vi "3_Axis_magmeter_MAIN.vi"() -> ()   [LabVIEW 2013]
doc: "Программа для обработки и визуализации трех компонент магнитного поля прибора, разработаного инженерами НЭОиКН ЛФВЭ ОИЯИ 2014"
uses:
  <vilib>/Utility/error.llb/DialogType.ctl
  <vilib>/Instr/_visa.llb/Select Event Type.ctl
  <vilib>/Instr/_visa.llb/VISA Configure Serial Port (Instr).vi
panel:
  in  "stop":bool
  out "Sens_con_status":bool caption="Датчик не подключен"
  out "Dx Sum":u64
  in  "Порт":refnum<visa-resource-name>="?"
  out "Соединение":bool
  out "i":i32
  in  "number of data sample":u64
  out "String 2":string
  out "String":string
  in  "Автосохранение":bool
  in  "Интервал [сек.]":u32=5 min=1 max=30000 step=1
  in  "Маркеры":bool
  out "Table num index":u32
  in  "Удалить измерение":bool
  in  "RXd number":u64
  in  "Dz, мм":u64=5 min=1
  in  "зафиксировать измерение":bool
  in  "Измерений":u16=100
  in  "Очистить историю":bool
  in  "H макс":dbl=8.0 format="%#.1f"
  in  "H мин":dbl=-8.0 format="%#.1f"
  in  "Уст. ноль":bool
  in  "Сохранен!":bool
  in  "Plot.Visible Z":bool
  out "By":dbl format="%04.1f"
  out "Bz":dbl format="%04.1f"
  in  "Plot.Visible X":bool
  out "Bx":dbl format="%04.1f"
  in  "Plot.Visible Y":bool
  in  "Графики толще":bool=TRUE
  in  "Стоп":bool
  out "Магнитные измерения":T1(graph)
  in  "Measurment Fl":bool
  out "Сохраненные измерения":string[][](table)
  out "Путь к файлу":path
  # "Гаусс"
  # "на графике"
  # "Результаты\nизмерений"
  # "ГС"
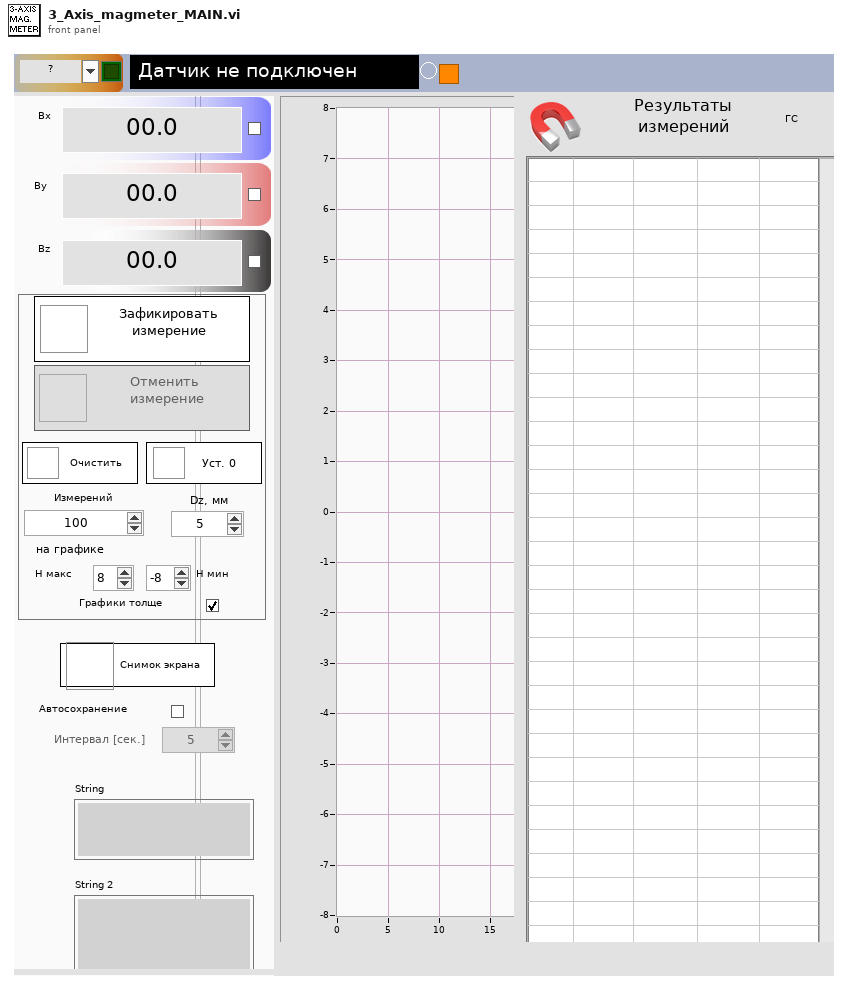
[diagram p1: front panel]
types:
  T1 = cluster{"X":dbl, "Y":dbl, "Z":dbl, "Active Plot":dbl}[]
  T2 = cluster{"Value":dbl, "Value":dbl, "Value":dbl, "Active Plot":dbl}
  T3 = cluster{"Value":dbl, "Value":dbl, "Value":dbl, "X":dbl}
  T4 = cluster{"Value":dbl, "Value":dbl, "Value":dbl, "X":dbl}[]
  T5 = typedef "imagedata.ctl" = cluster{"image type":i32, "image depth":i32, "image":u8[], "mask":u8[], "colors":u32[], "Rectangle":cluster{"left":i16, "top":i16, "right":i16, "bottom":i16}}
  T6 = typedef "Select Event Type.ctl" = u32
  T7 = typedef "DialogType.ctl" = u16
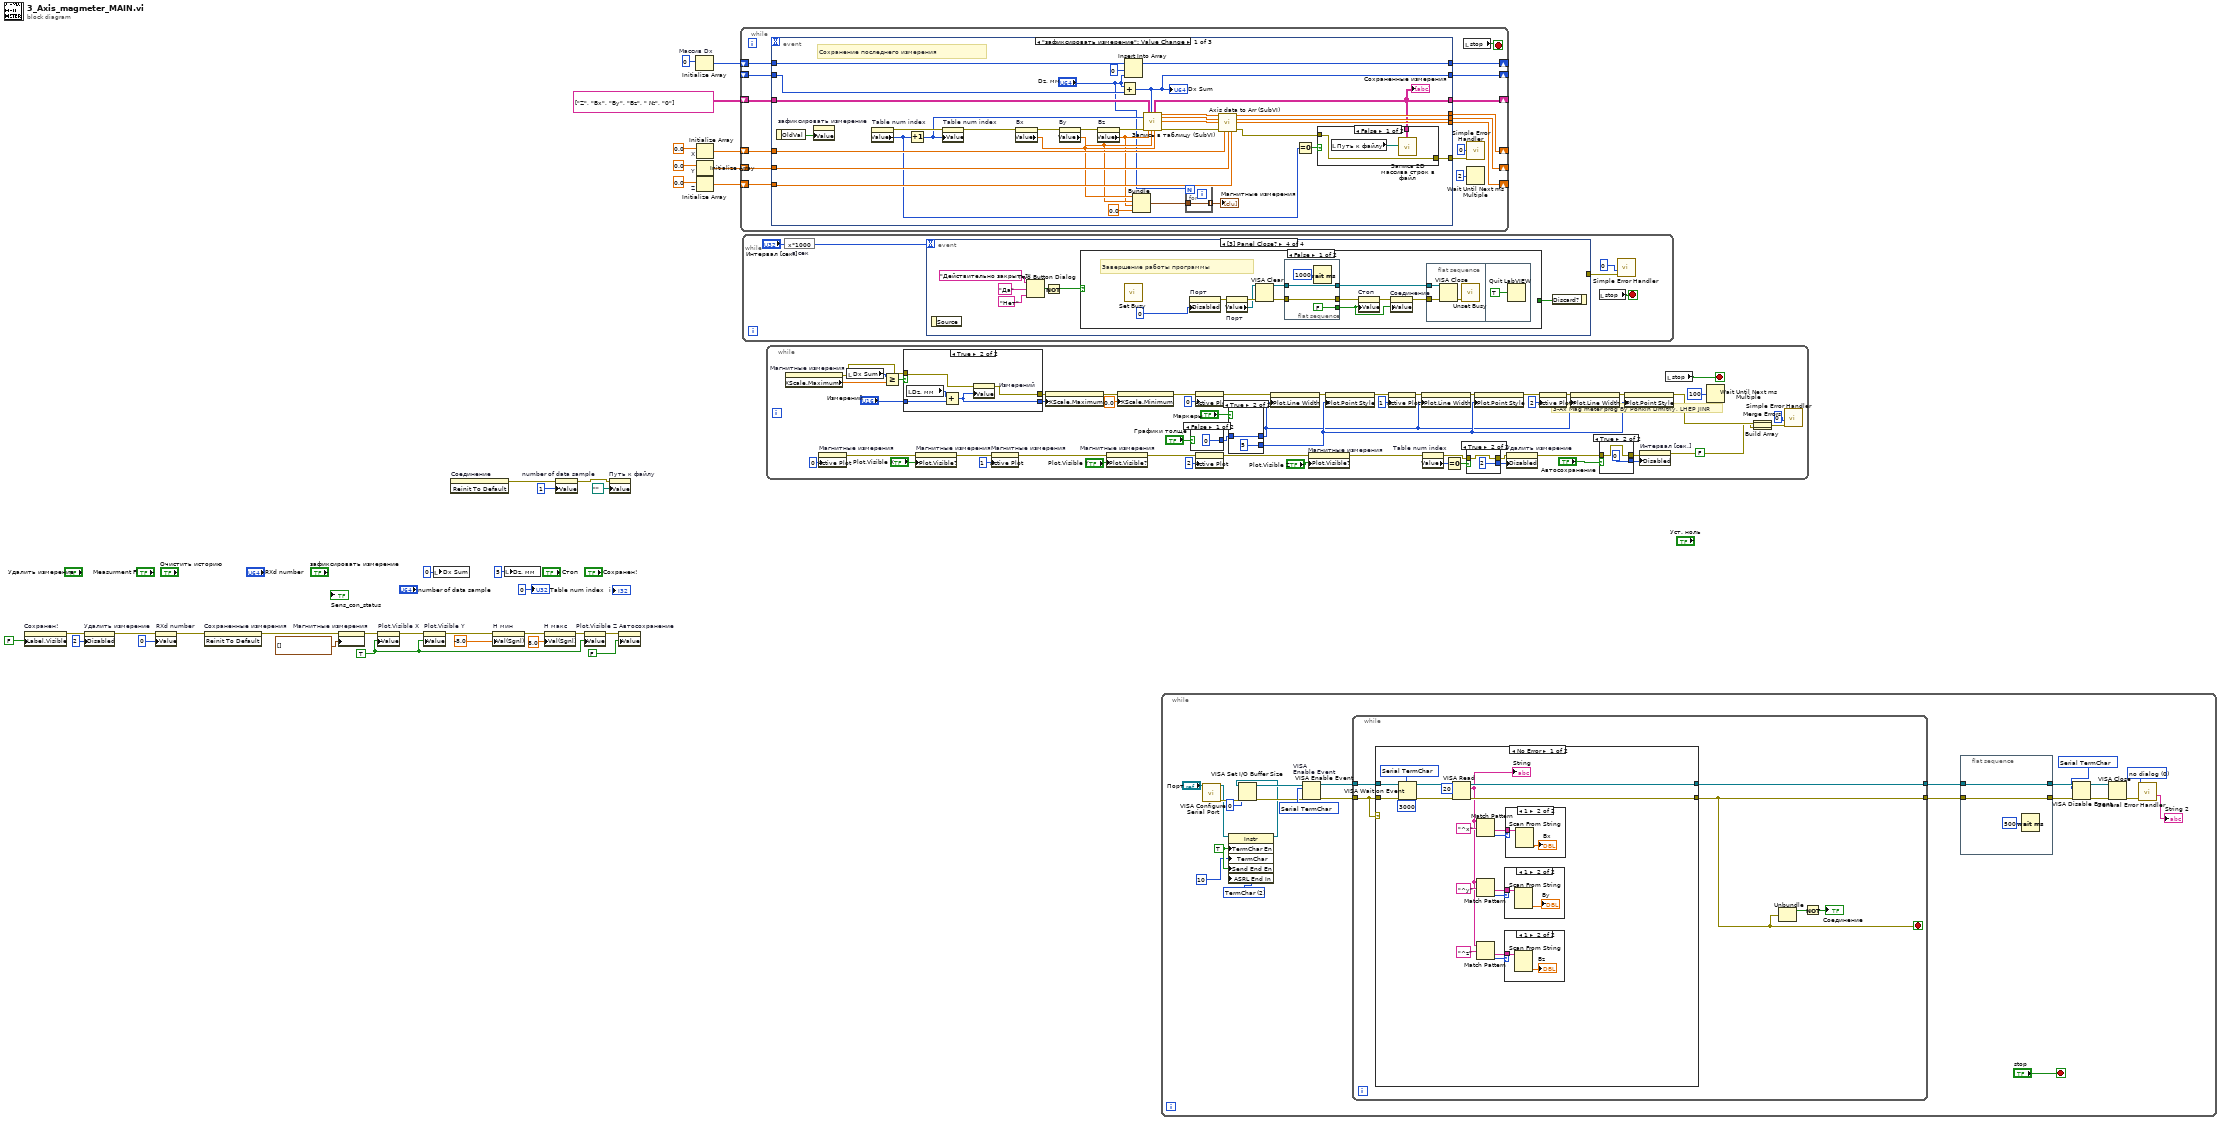
[diagram p0: block diagram]
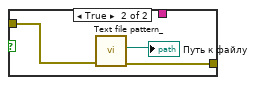
[diagram p6: hidden frame]
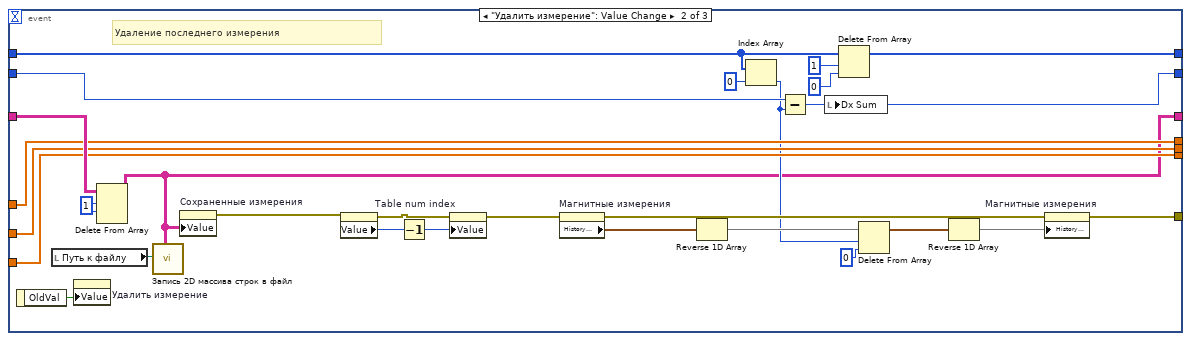
[diagram p7: hidden frame]
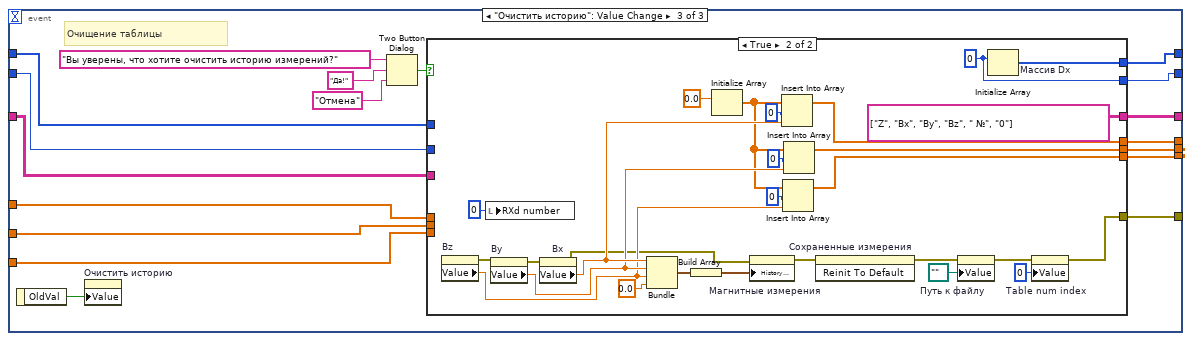
[diagram p8: hidden frame]
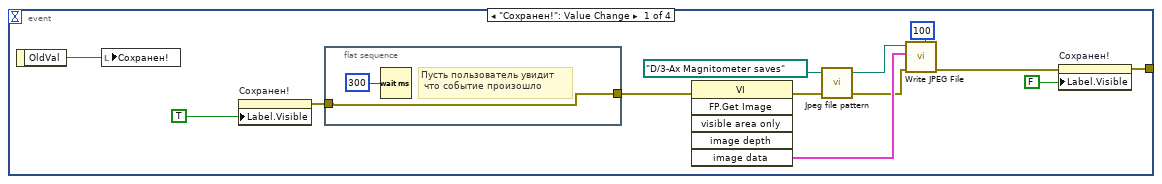
[diagram p10: hidden frame]
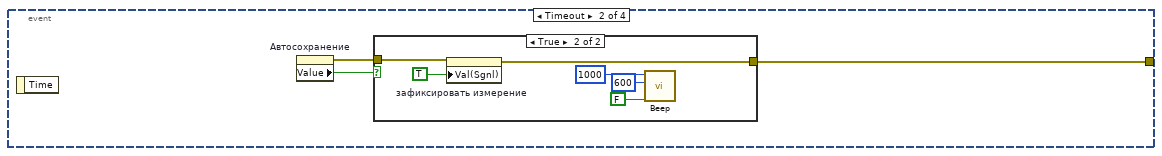
[diagram p11: hidden frame]
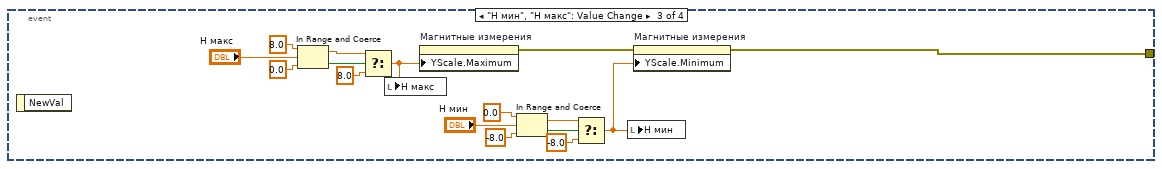
[diagram p13: hidden frame]
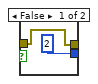
[diagram p15: hidden frame]
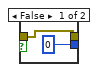
[diagram p16: hidden frame]
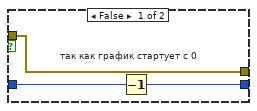
[diagram p17: hidden frame]
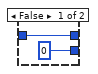
[diagram p18: hidden frame]
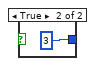
[diagram p19: hidden frame]
diagram:
  (unwired) FALSE
  w23 = TRUE ("Plot.Visible X")
  # "3-Ax Mag meter prog By Ponkin Dmitriy, LHEP JINR"
  n1 = property on="Сохранен!" class="Bool (strict)"("Label.Visible"=FALSE) -> (error out=w14:errorcluster)  [unwired: 2 in, 1 out]
  n2 = property on="Удалить измерение" class="Bool (strict)"(error in=w14, "Disabled"=u8 2) -> (error out=w12:errorcluster)  [unwired: 1 in, 1 out]
  n3 = property on="RXd number" class="DigNum (strict)"(error in=w12, "Value"=u64 0 ("RXd number")) -> (error out=w11:errorcluster)  [unwired: 1 in, 1 out]
  n4 = invoke on="Сохраненные измерения" class="Tbl (strict)" method="Reinit To Default"(error in=w11) -> (error out=w10:errorcluster)  [unwired: 2 in, 2 out]
  n5 = property on="Магнитные измерения" class="WFChart (strict)"(error in=w10, "History Data"=T1 []) -> (error out=w8:errorcluster)  [unwired: 1 in, 1 out]
  n6 = property on="Plot.Visible X" class="Bool (strict)"(error in=w8, "Value"=w23) -> (error out=w6:errorcluster)  [unwired: 1 in, 1 out]
  n7 = property on="Plot.Visible Y" class="Bool (strict)"(error in=w6, "Value"=w23) -> (error out=w17:errorcluster)  [unwired: 1 in, 1 out]
  n8 = local write "Dx Sum"(u64 0 ("Dx Sum")) -> ()
  n9 = invoke on="Соединение" class="Bool (strict)" method="Reinit To Default"() -> (error out=w2:errorcluster)  [unwired: 3 in, 2 out]
  n10 = property on="H мин" class="DigNum (strict)"(error in=w17, "Val(Sgnl)"=-8.0 ("Value (Signaling)")) -> (error out=w19:errorcluster)  [unwired: 1 in, 1 out]
  n11 = local write "Dz, мм"(u64 5 ("Dz, мм")) -> ()
  n12 = property on="H макс" class="DigNum (strict)"(error in=w19, "Val(Sgnl)"=8.0 ("Value (Signaling)")) -> (error out=w20:errorcluster)  [unwired: 1 in, 1 out]
  n13 = property on="number of data sample" class="DigNum (strict)"(error in=w2, "Value"=u64 1 ("number of data sample")) -> (error out=w4:errorcluster)  [unwired: 1 in, 1 out]
  n14 = property on="Plot.Visible Z" class="Bool (strict)"(error in=w20, "Value"=w23) -> (error out=w24:errorcluster)  [unwired: 1 in, 1 out]
  n15 = property on="Путь к файлу" class="Path"(error in=w4, "Value"=path "" ("Путь к файлу")) -> ()  [unwired: 1 in, 2 out]
  n16 = property on="Автосохранение" class="Bool (strict)"(error in=w24, "Value"=FALSE ("Plot.Visible X")) -> ()  [unwired: 1 in, 2 out]
  n17 = Initialize Array "Массив Dx"(u64 0 ("element")) -> (w26:u64[])  [unwired: 1 out]
  n18 = Initialize Array "X"(0.0 ("element")) -> (w32:dbl[])  [unwired: 1 out]
  n19 = Initialize Array "Y"(0.0 ("element")) -> (w29:dbl[])  [unwired: 1 out]
  n20 = Initialize Array "Z"(0.0 ("element")) -> (w28:dbl[])  [unwired: 1 out]
  n21 = while {
    shift-right: [w50] -> _
    shift-left: string[][] [["Z", "Bx", "By", "Bz", " №", "0"]] ("Сохраненные измерения") -> [w49]
    shift-right: [w47] -> _
    shift-left: w32 -> [w48]
    shift-right: [w41] -> _
    shift-left: w28 -> [w43]
    shift-right: [w42] -> _
    shift-left: w29 -> [w44]
    shift-right: [w40] -> _
    shift-left: w26 -> [w39]
    shift-right: [w38] -> _
    shift-left: _ -> [w37]
    stop <- w35 stop-if-true
    n22 = event shown="[0] \"зафиксировать измерение\": Value Change" {
      selector: _ -> [_ _ _]
      dyn-events: _ -> [_ _ _]
      timeout: _ -> [_ _ _]
      tunnel: w49 -> [w69 w118 w136]
      tunnel: [w51 w104 w137] -> w46
      tunnel: [w54 w94 w138] -> w50
      tunnel: w48 -> [w76 w116 w130]
      tunnel: [w73 w116 w131] -> w47
      tunnel: w44 -> [w75 w114 w129]
      tunnel: w43 -> [w74 w113 w128]
      tunnel: [w72 w113 w126] -> w41
      tunnel: [w71 w114 w127] -> w42
      tunnel: [w64 w101 w125] -> w40
      tunnel: w39 -> [w67 w96 w122]
      tunnel: [w66 w97 w124] -> w38
      tunnel: w37 -> [w65 w99 w123]
      event "зафиксировать измерение": Value Change {
        # "Сохранение последнего измерения"
        n23 = event-data() -> ("OldVal"=w61:bool)  [unwired: 1 out]
        n24 = property on="зафиксировать измерение" class="Bool (strict)"("Value"=w61) -> ()  [unwired: 2 in, 2 out]
        n25 = property on="Table num index" class="DigNum (strict)"() -> (error out=w85:errorcluster, "Value"=w53:u32)  [unwired: 2 in, 1 out]
        n26 = Increment(x=w53) -> (x+1=w70:u32)
        n27 = property on="Table num index" class="DigNum (strict)"(error in=w85, "Value"=w70) -> (error out=w82:errorcluster)  [unwired: 1 in, 1 out]
        n28 = property on="Bx" class="DigNum (strict)"(error in=w82) -> (error out=w84:errorcluster, "Value"=w60:dbl)  [unwired: 1 in, 1 out]
        n29 = property on="By" class="DigNum (strict)"(error in=w84) -> (error out=w83:errorcluster, "Value"=w59:dbl)  [unwired: 1 in, 1 out]
        n30 = property on="Bz" class="DigNum (strict)"(error in=w83) -> (error out=w81:errorcluster, "Value"=w58:dbl)  [unwired: 1 in, 1 out]
        n31 = Add(x="Dz, мм", y=w65) -> (x+y=w66:u64)
        "Dx Sum" <- w66
        n32 = Insert Into Array "Insert Into Array"(array=w67, index=0, new element="Dz, мм") -> (w64:u64[])
        n33 = Bundle("Value"=w60, "Value"=w59, "Value"=w58, "Active Plot"=0.0) -> (w63:T2)  [unwired: 1 out]
        n34 = call "Запись в таблицу (SubVI).vi"("data num"=w70, "error in"=w81, "String Arr in"=w69, "Z axis data"=w58, "Шаг измерений"=w66, "Y axis data"=w59, "X axis data"=w60) -> ("String Arr out"=w54:string[][], "X axis data out"=w79:dbl, "Y axis data out"=w78:dbl, "Z axis data out"=w77:dbl, "error out"=w80:errorcluster)  [unwired: 5 in, 3 out]
        "Сохраненные измерения" <- w54
        n35 = for {
          N: "Dz, мм" -> [_]
          tunnel: [w92] -> w56 mode=indexing
          tunnel: w63 -> [w92]
        }
        "Магнитные измерения" <- w56
        n36 = call "Axis data to Arr (SubVI).vi"("new X element"=w79, "new Y element"=w78, "new Z element"=w77, "error in"=w80, "X Arr in"=w76, "Y Arr in"=w75, "Z Arr in"=w74) -> ("X Arr Out"=w73:dbl[], "Y Arr Out"=w71:dbl[], "Z Arr Out"=w72:dbl[], "error out"=w52:errorcluster)  [unwired: 5 out]
        n37 = Equal To 0?(x=w53) -> (x = 0?=w55:bool)
        n38 = case shown="False" w55 {
          tunnel: w54 -> [w88 _]
          tunnel: w52 -> [w86 w90]
          tunnel: [w86 w89] -> w51
          frame False {
            n39 = local read "Путь к файлу"() -> (w87:path)
            n40 = call "Запись 2D массива строк в файл.vi"("путь к файлу"=w87, "2-D массив строк для записи"=w88) -> ()  [unwired: 2 in, 16 out]
          }
          frame True {
            n41 = call "Text file pattern_.vi"("error in"=w90) -> ("error out"=w89:errorcluster, "путь к файлу"=→"Путь к файлу":path)  [unwired: 9 out]
          }
        }
      }
      event "Удалить измерение": Value Change {
        w117 = 1 ("length")
        # "Удаление последнего измерения"
        n42 = event-data() -> ("OldVal"=w95:bool)  [unwired: 1 out]
        n43 = local read "Путь к файлу"() -> (w93:path)
        n44 = property on="Удалить измерение" class="Bool (strict)"("Value"=w95) -> ()  [unwired: 2 in, 2 out]
        n45 = Delete From Array "Delete From Array"(array=w118, length=w117, index (row)=w117) -> (array with subset deleted=w94:string[][])  [unwired: 1 in, 1 out]
        n46 = call "Запись 2D массива строк в файл.vi"("путь к файлу"=w93, "2-D массив строк для записи"=w94) -> ()  [unwired: 2 in, 16 out]
        n47 = property on="Сохраненные измерения" class="Tbl (strict)"("Value"=w94) -> (error out=w105:errorcluster)  [unwired: 2 in, 1 out]
        n48 = property on="Table num index" class="DigNum (strict)"(error in=w105) -> (error out=w115:errorcluster, "Value"=w120:u32)  [unwired: 1 in, 1 out]
        n49 = Decrement(x=w120) -> (x-1=w119:u32)
        n50 = property on="Table num index" class="DigNum (strict)"(error in=w115, "Value"=w119) -> (error out=w106:errorcluster)  [unwired: 1 in, 1 out]
        n51 = property on="Магнитные измерения" class="WFChart (strict)"(error in=w106) -> (error out=w107:errorcluster, "History Data"=w111:T1)  [unwired: 1 in, 1 out]
        n52 = Reverse 1D Array(array=w111) -> (reversed array=w110:T1)
        n53 = Index Array "Index Array"(array=w96, index=0) -> (element=w98:u64)
        n54 = Subtract(x=w99, y=w98) -> (x-y=w97:u64)
        n55 = local write "Dx Sum"(w97) -> ()
        n56 = Delete From Array "Delete From Array"(array=w96, length=1, index=0 ("length")) -> (array with subset deleted=w101:u64[])  [unwired: 1 out]
        n57 = Delete From Array "Delete From Array"(array=w110, length=w98, index=0 ("length")) -> (array with subset deleted=w108:T1)  [unwired: 1 out]
        n58 = Reverse 1D Array(array=w108) -> (reversed array=w109:T1)
        n59 = property on="Магнитные измерения" class="WFChart (strict)"(error in=w107, "History Data"=w109) -> (error out=w104:errorcluster)  [unwired: 1 in, 1 out]
      }
      event "Очистить историю": Value Change {
        # "Очищение таблицы"
        n60 = event-data() -> ("OldVal"=w121:bool)  [unwired: 1 out]
        n61 = property on="Очистить историю" class="Bool (strict)"("Value"=w121) -> ()  [unwired: 2 in, 2 out]
        n62 = Two Button Dialog(message="Вы уверены, что хотите очистить историю измерений?", 1:"Отмена" ("T button name (\"OK\")"), 2:"Да!" ("T button name (\"OK\")")) -> (T button?=w132:bool)
        n63 = case shown="True" w132 {
          tunnel: [w144 string[][] [["Z", "Bx", "By", "Bz", " №", "0"]] ("Сохраненные измерения")] -> w138
          tunnel: [_ w151] -> w137
          tunnel: w136 -> [w144 _]
          tunnel: [w143 w164] -> w131
          tunnel: w130 -> [w143 _]
          tunnel: w129 -> [w142 _]
          tunnel: w128 -> [w141 _]
          tunnel: [w142 w159] -> w127
          tunnel: [w141 w157] -> w126
          tunnel: w122 -> [w140 _]
          tunnel: [w140 w150] -> w125
          tunnel: [w139 w149] -> w124
          tunnel: w123 -> [w139 _]
          frame False {
          }
          frame True {
            w149 = u64 0 ("element")
            n64 = property on="Bz" class="DigNum (strict)"() -> (error out=w154:errorcluster, "Value"=w156:dbl)  [unwired: 2 in, 1 out]
            n65 = local write "RXd number"(u64 0 ("RXd number")) -> ()
            n66 = property on="By" class="DigNum (strict)"(error in=w154) -> (error out=w153:errorcluster, "Value"=w160:dbl)  [unwired: 1 in, 1 out]
            n67 = property on="Bx" class="DigNum (strict)"(error in=w153) -> (error out=w152:errorcluster, "Value"=w161:dbl)  [unwired: 1 in, 1 out]
            n68 = Bundle("Value"=w161, "Value"=w160, "Value"=w156, "X"=0.0) -> (w167:T3)  [unwired: 1 out]
            n69 = Build Array(w167) -> (w162:T4)
            n70 = Initialize Array(0.0 ("element")) -> (w155:dbl[])  [unwired: 1 out]
            n71 = property on="Магнитные измерения" class="WFChart (strict)"(error in=w152, "History Data"=w162) -> (error out=w169:errorcluster)  [unwired: 1 in, 1 out]
            n72 = Insert Into Array(array=w155, index=0, new element=w161) -> (w164:dbl[])
            n73 = Insert Into Array(array=w155, index=0, new element=w156) -> (w157:dbl[])
            n74 = Insert Into Array(array=w155, index=0, new element=w160) -> (w159:dbl[])
            n75 = invoke on="Сохраненные измерения" class="Tbl (strict)" method="Reinit To Default"(error in=w169) -> (error out=w146:errorcluster)  [unwired: 2 in, 2 out]
            n76 = property on="Путь к файлу" class="Path"(error in=w146, "Value"=path "" ("Путь к файлу")) -> (error out=w145:errorcluster)  [unwired: 1 in, 1 out]
            n77 = Initialize Array "Массив Dx"(w149) -> (w150:u64[])  [unwired: 1 out]
            n78 = property on="Table num index" class="DigNum (strict)"(error in=w145, "Value"=u32 0 ("Table num index")) -> (error out=w151:errorcluster)  [unwired: 1 in, 1 out]
          }
        }
      }
    }
    n79 = local read "stop"() -> (w35:bool)
    n80 = call <vilib>:"Simple Error Handler.vi"("type of dialog (OK msg:1)"=u32 0 ("Table num index"), "error in (no error)"=w46) -> ()  [unwired: 8 out]
    n81 = Wait Until Next ms Multiple(millisecond multiple=u32 2) -> ()  [unwired: 1 out]
  }
  n82 = while {
    stop <- w172 stop-if-true
    n83 = expression code="x*1000" "в сек"("Интервал [сек.]") -> (w173:u32)
    n84 = event shown="[3] Panel Close?" {
      selector: _ -> [_ _ _ _]
      dyn-events: _ -> [_ _ _ _]
      timeout: w173 -> [_ _ _ _]
      tunnel: [w183 w194 w202 _] -> w176
      event "Сохранен!": Value Change {
        n85 = event-data() -> ("OldVal"=w184:bool)  [unwired: 1 out]
        n86 = local write "Сохранен!"(w184) -> ()
        n87 = property on="Сохранен!" class="Bool (strict)"("Label.Visible"=TRUE) -> (error out=w178:errorcluster)  [unwired: 2 in, 1 out]
        n88 = flat-sequence {
          tunnel: [w190] -> w179
          tunnel: w178 -> [w190]
          frame #0 {
            # "Пусть пользователь увидит\n что событие произошло"
            n89 = Wait (ms)(milliseconds to wait=u32 300) -> ()  [unwired: 1 out]
          }
        }
        n90 = invoke class="VI" method="FP.Get Image"(error in=w179) -> (error out=w187:errorcluster, "image data"=w188:T5)  [unwired: 5 in, 4 out]
        n91 = call "Jpeg file pattern.vi"("path"=path "D:/3-Ax Magnitometer saves" ("path (use dialog)"), "error in"=w187) -> ("path to JPG file"=w186:path, "error out"=w185:errorcluster)  [unwired: 6 out]
        n92 = call <vilib>:"Write JPEG File.vi"("quality (80)"=100, "error in (no error)"=w185, "image data"=w188, "path to JPEG file"=w186) -> ("error out"=w182:errorcluster)  [unwired: 7 out]
        n93 = property on="Сохранен!" class="Bool (strict)"(error in=w182, "Label.Visible"=FALSE) -> (error out=w183:errorcluster)  [unwired: 1 in, 1 out]
      }
      event Timeout {
        n94 = event-data() -> ()  [unwired: 2 out]
        n95 = property on="Автосохранение" class="Bool (strict)"() -> (error out=w192:errorcluster, "Value"=w193:bool)  [unwired: 2 in, 1 out]
        n96 = case shown="True" w193 {
          tunnel: [w195 w200] -> w194
          tunnel: w192 -> [w195 w199]
          frame False {
          }
          frame True {
            n97 = property on="зафиксировать измерение" class="Bool (strict)"(error in=w199, "Val(Sgnl)"=TRUE ("Value (Signaling)")) -> (error out=w200:errorcluster)  [unwired: 1 in, 1 out]
            n98 = call <vilib>:"Beep.vi"("use system alert? (T)"=FALSE, "duration (msec)"=u32 600, "frequency (Hz)"=u32 1000 ("duration (msec)")) -> ()  [unwired: 9 out]
          }
        }
      }
      event "H мин", "H макс": Value Change {
        n99 = event-data() -> ()  [unwired: 2 out]
        n100 = In Range and Coerce(upper limit=8.0, x="H макс", lower limit=0.0) -> (coerced(x)=w213:dbl, In Range?=w215:bool)
        n101 = Select(t=w213, s=w215, f=8.0) -> (s? t:f=w205:dbl)
        n102 = local write "H макс"(w205) -> ()
        n103 = property on="Магнитные измерения" class="WFChart (strict)"("YScale.Maximum"=w205) -> (error out=w203:errorcluster)  [unwired: 2 in, 1 out]
        n104 = In Range and Coerce(upper limit=0.0, x="H мин", lower limit=-8.0) -> (coerced(x)=w211:dbl, In Range?=w209:bool)
        n105 = Select(t=w211, s=w209, f=-8.0) -> (s? t:f=w204:dbl)
        n106 = local write "H мин"(w204) -> ()
        n107 = property on="Магнитные измерения" class="WFChart (strict)"(error in=w203, "YScale.Minimum"=w204) -> (error out=w202:errorcluster)  [unwired: 1 in, 1 out]
      }
      event Panel Close? {
        n108 = event-data() -> ()  [unwired: 2 out]
        n109 = Two Button Dialog(message="Действительно закрыть?", 1:"Нет", 2:"Да") -> (T button?=w220:bool)
        n110 = Not(x=w220) -> (.not. x?=w219:bool)
        n111 = case shown="False" w219 {
          selector: w219 -> [_ w243]
          tunnel: [_ w243] -> w218
          frame False {
            # "Завершение работы программы"
            n112 = call <vilib>:"Set Busy.vi"() -> ()  [unwired: 4 in, 8 out]
            n113 = property on="Порт" class="VISAName"("Disabled"=u8 0) -> (error out=w224:errorcluster)  [unwired: 2 in, 1 out]
            n114 = property on="Порт" class="VISAName"(error in=w224) -> (error out=w226:errorcluster, "Value"=w225:refnum<visa-resource-name>)  [unwired: 1 in, 1 out]
            n115 = VISA Clear(VISA resource name=w225, error in (no error)=w226) -> (VISA resource name out=w234:refnum<visa-resource-name>, error out=w233:errorcluster)
            n116 = flat-sequence {
              tunnel: w234 -> [w237]
              tunnel: [w237] -> w230
              tunnel: [w236] -> w228
              tunnel: w233 -> [w236]
              tunnel: [FALSE ("Visible")] -> w227
              frame #0 {
                n117 = Wait (ms)(milliseconds to wait=u32 1000) -> ()  [unwired: 1 out]
              }
            }
            n118 = property on="Стоп" class="Bool (strict)"(error in=w228, "Value"=w227) -> (error out=w229:errorcluster)  [unwired: 1 in, 1 out]
            n119 = property on="Соединение" class="Bool (strict)"(error in=w229, "Value"=w227) -> (error out=w231:errorcluster)  [unwired: 1 in, 1 out]
            n120 = flat-sequence {
              tunnel: w231 -> [w241]
              tunnel: w230 -> [w240]
              frame #0 {
                n121 = VISA Close(VISA resource name=w240, error in (no error)=w241) -> (error out=w239:errorcluster)
                n122 = call <vilib>:"Unset Busy.vi"("error in (no error)"=w239) -> ()  [unwired: 1 in, 10 out]
              }
              frame #1 {
                n123 = Quit LabVIEW(quit? (T)=TRUE ("stop? (T)")) -> ()
              }
            }
          }
          frame True {
          }
        }
        n124 = event-data("Discard?"=w218) -> ()  [unwired: 1 in, 1 out]
      }
    }
    n125 = local read "stop"() -> (w172:bool)
    n126 = call <vilib>:"Simple Error Handler.vi"("type of dialog (OK msg:1)"=u32 0 ("Table num index"), "error in (no error)"=w176) -> ()  [unwired: 8 out]
  }
  n127 = while {
    stop <- w244 stop-if-true
    n128 = property on="Магнитные измерения" class="WFChart (strict)"() -> (error out=w260:errorcluster, "XScale.Maximum"=w265:dbl)  [unwired: 2 in, 1 out]
    n129 = property on="Магнитные измерения" class="WFChart (strict)"("Active Plot"=u32 0) -> (error out=w270:errorcluster)  [unwired: 2 in, 1 out]
    n130 = local read "Dx Sum"() -> (w267:u64)
    n131 = Greater Or Equal?(x=w267, y=w265) -> (x >= y?=w266:bool)
    n132 = case shown="True" w266 {
      tunnel: [w308 w312] -> w268
      tunnel: "Измерений" -> [w307 w311]
      tunnel: w260 -> [w306 w310]
      tunnel: [w306 w309] -> w259
      frame False {
        n133 = Decrement "так как график стартует с 0"(x=w307) -> (x-1=w308:u16)
      }
      frame True {
        n134 = local read "Dz, мм"() -> (w313:u64)
        n135 = Add(x=w313, y=w311) -> (x+y=w312:u64)
        n136 = property on="Измерений" class="DigNum (strict)"(error in=w310, "Value"=w312) -> (error out=w309:errorcluster)  [unwired: 1 in, 1 out]
      }
    }
    n137 = property on="Магнитные измерения" class="WFChart (strict)"(error in=w270, "Plot.Visible?"="Plot.Visible X") -> (error out=w291:errorcluster)  [unwired: 1 in, 1 out]
    n138 = property on="Магнитные измерения" class="WFChart (strict)"(error in=w291, "Active Plot"=u32 1) -> (error out=w289:errorcluster)  [unwired: 1 in, 1 out]
    n139 = property on="Магнитные измерения" class="WFChart (strict)"(error in=w259, "XScale.Maximum"=w268) -> (error out=w271:errorcluster)  [unwired: 1 in, 1 out]
    n140 = property on="Магнитные измерения" class="WFChart (strict)"(error in=w289, "Plot.Visible?"="Plot.Visible Y") -> (error out=w273:errorcluster)  [unwired: 1 in, 1 out]
    n141 = property on="Магнитные измерения" class="WFChart (strict)"(error in=w271, "XScale.Minimum"=0.0 ("X Scale.Range:Minimum")) -> (error out=w269:errorcluster)  [unwired: 1 in, 1 out]
    n142 = case shown="False" "Графики толще" {
      tunnel: [u8 0 ("Plot.Line Width") u8 3 ("Plot.Line Width")] -> w277
      frame False {
      }
      frame True {
      }
    }
    n143 = property on="Магнитные измерения" class="WFChart (strict)"(error in=w269, "Active Plot"=u32 0) -> (error out=w272:errorcluster)  [unwired: 1 in, 1 out]
    n144 = property on="Магнитные измерения" class="WFChart (strict)"(error in=w273, "Active Plot"=u32 2) -> (error out=w293:errorcluster)  [unwired: 1 in, 1 out]
    n145 = case shown="True" "Маркеры" {
      tunnel: [w315 w317] -> w263
      tunnel: w277 -> [w315 w317]
      tunnel: [u8 0 ("Plot.Line Width") u8 5 ("Plot.Line Width")] -> w275
      frame False {
      }
      frame True {
      }
    }
    n146 = property on="Магнитные измерения" class="WFChart (strict)"(error in=w272, "Plot.Line Width"=w263) -> (error out=w281:errorcluster)  [unwired: 1 in, 1 out]
    n147 = property on="Магнитные измерения" class="WFChart (strict)"(error in=w293, "Plot.Visible?"="Plot.Visible Z") -> (error out=w258:errorcluster)  [unwired: 1 in, 1 out]
    n148 = property on="Магнитные измерения" class="WFChart (strict)"(error in=w281, "Plot.Point Style"=w275) -> (error out=w282:errorcluster)  [unwired: 1 in, 1 out]
    n149 = property on="Магнитные измерения" class="WFChart (strict)"(error in=w282, "Active Plot"=u32 1) -> (error out=w287:errorcluster)  [unwired: 1 in, 1 out]
    n150 = property on="Магнитные измерения" class="WFChart (strict)"(error in=w287, "Plot.Line Width"=w263) -> (error out=w279:errorcluster)  [unwired: 1 in, 1 out]
    n151 = property on="Table num index" class="DigNum (strict)"(error in=w258) -> (error out=w251:errorcluster, "Value"=w256:u32)  [unwired: 1 in, 1 out]
    n152 = Equal To 0?(x=w256) -> (x = 0?=w255:bool)
    n153 = case shown="True" w255 {
      tunnel: [u32 0 ("Table num index") u32 2 ("Table num index")] -> w254
      tunnel: w251 -> [w302 w304]
      tunnel: [w302 w304] -> w250
      frame False {
      }
      frame True {
      }
    }
    n154 = property on="Магнитные измерения" class="WFChart (strict)"(error in=w279, "Plot.Point Style"=w275) -> (error out=w280:errorcluster)  [unwired: 1 in, 1 out]
    n155 = property on="Удалить измерение" class="Bool (strict)"(error in=w250, "Disabled"=w254) -> (error out=w247:errorcluster)  [unwired: 1 in, 1 out]
    n156 = property on="Магнитные измерения" class="WFChart (strict)"(error in=w280, "Active Plot"=u32 2) -> (error out=w284:errorcluster)  [unwired: 1 in, 1 out]
    n157 = property on="Магнитные измерения" class="WFChart (strict)"(error in=w284, "Plot.Line Width"=w263) -> (error out=w278:errorcluster)  [unwired: 1 in, 1 out]
    n158 = case shown="True" "Автосохранение" {
      tunnel: [u8 2 ("Plot.Line Width") u8 0 ("Plot.Line Width")] -> w253
      tunnel: w247 -> [w298 w300]
      tunnel: [w298 w300] -> w252
      frame False {
      }
      frame True {
      }
    }
    n159 = property on="Магнитные измерения" class="WFChart (strict)"(error in=w278, "Plot.Point Style"=w275) -> (error out=w249:errorcluster)  [unwired: 1 in, 1 out]
    n160 = property on="Интервал [сек.]" class="DigNum (strict)"(error in=w252, "Disabled"=w253) -> (error out=w246:errorcluster)  [unwired: 1 in, 1 out]
    n161 = local read "stop"() -> (w244:bool)
    n162 = Wait Until Next ms Multiple(millisecond multiple=u32 100) -> ()  [unwired: 1 out]
    n163 = Build Array(w249, w246) -> (w245:errorcluster[])
    n164 = Merge Errors(w245) -> (w261:errorcluster)
    n165 = call <vilib>:"Simple Error Handler.vi"("type of dialog (OK msg:1)"=u32 0 ("Table num index"), "error in (no error)"=w261) -> ()  [unwired: 8 out]
  }
  n166 = while {
    stop <- "stop" stop-if-true
    w321 = T6 1073684516 items=["Service Request"=1073684491, "Trigger"=3221168138, "Clear"=1073684493, "VXI Signal"=1073684512, "VXI/VME Interrupt"=3221168161, "VXI/VME Sysfail"=1073684509, "VXI/VME Sysreset"=1073684510, "GPIB CIC"=1073684498, "GPIB Talk"=1073684499, "GPIB Listen"=1073684500, "PXI Interrupt"=1073684514, "Serial Break"=1073684515, "Serial TermChar"=1073684516, "Serial CTS"=1073684521, "Serial DSR"=1073684522, "Serial DCD"=1073684524, "Serial RI"=1073684526, "Serial Character"=1073684533, "USB Interrupt"=1073684535, "All Enabled"=1073709055] ("Event Type")
    w327 = u16 2 items=["None", "Last Bit", "TermChar"] ("Serial Settings:End Mode for Reads")
    w328 = TRUE ("Message Based Settings:Termination Character Enable")
    w335 = T6 1073684516 items=["Service Request"=1073684491, "Trigger"=3221168138, "Clear"=1073684493, "VXI Signal"=1073684512, "VXI/VME Interrupt"=3221168161, "VXI/VME Sysfail"=1073684509, "VXI/VME Sysreset"=1073684510, "GPIB CIC"=1073684498, "GPIB Talk"=1073684499, "GPIB Listen"=1073684500, "PXI Interrupt"=1073684514, "Serial Break"=1073684515, "Serial TermChar"=1073684516, "Serial CTS"=1073684521, "Serial DSR"=1073684522, "Serial DCD"=1073684524, "Serial RI"=1073684526, "Serial Character"=1073684533, "USB Interrupt"=1073684535, "All Enabled"=1073709055] ("Event Type")
    w337 = T7 0 items=["no dialog", "OK message", "continue or stop message", "OK message + warnings", "continue/stop + warnings"] ("type of dialog (OK msg:1)")
    n167 = call-poly "VISA Configure Serial Port"("VISA resource name"="Порт") -> ("VISA resource name out"=w330:refnum<visa-resource-name>, "error out"=w334:errorcluster)  [unwired: 5 in, 8 out]
    n168 = property class="Instr"(reference=w330, "TermChar En"=w328, "TermChar"=u32 10 ("size (4096)"), "Send End En"=w328, "ASRL End In"=w327) -> (reference out=w329:refnum<visa-resource-name>)  [unwired: 1 in, 1 out]
    n169 = VISA Set I/O Buffer Size(VISA resource name=w329, size (4096)=u32 0, error in (no error)=w334) -> (VISA resource name out=w331:refnum<visa-resource-name>, error out=w332:errorcluster)  [unwired: 1 in]
    n170 = VISA Enable Event "VISA \nEnable Event"(8:w332, 10:w335, 11:w331) -> (0:w342:errorcluster, 3:w343:refnum<visa-resource-name>)  [unwired: 1 in]
    n171 = while {
      tunnel: w343 -> [w352]
      tunnel: w342 -> [w351]
      tunnel: [w350] -> w324
      tunnel: [w349] -> w322
      stop <- w349 stop-if-true
      n172 = case shown="No Error" w351 {
        tunnel: w352 -> [w371 w379]
        tunnel: w351 -> [w370 w378]
        tunnel: [w367 w379] -> w350
        tunnel: [w366 w378] -> w349
        frame No Error {
          w361 = T6 1073684516 items=["Service Request"=1073684491, "Trigger"=3221168138, "Clear"=1073684493, "VXI Signal"=1073684512, "VXI/VME Interrupt"=3221168161, "VXI/VME Sysfail"=1073684509, "VXI/VME Sysreset"=1073684510, "GPIB CIC"=1073684498, "GPIB Talk"=1073684499, "GPIB Listen"=1073684500, "PXI Interrupt"=1073684514, "Serial Break"=1073684515, "Serial TermChar"=1073684516, "Serial CTS"=1073684521, "Serial DSR"=1073684522, "Serial DCD"=1073684524, "Serial RI"=1073684526, "Serial Character"=1073684533, "USB Interrupt"=1073684535, "All Enabled"=1073709055] ("Event Type")
          n173 = VISA Wait on Event ("VISA Wait \non Event")(7:u32 3000 ("timeout (0)"), 8:w370, 10:w361, 11:w371) -> (0:w369:errorcluster, 3:w368:refnum<visa-resource-name>)  [unwired: 1 in, 2 out]
          n174 = VISA Read(VISA resource name=w368, byte count=u32 20, error in (no error)=w369) -> (VISA resource name out=w367:refnum<visa-resource-name>, read buffer=w353:string, error out=w366:errorcluster)  [unwired: 1 out]
          "String" <- w353
          n175 = Match Pattern(string=w353, regular expression="^y" ("Axis ID")) -> (after substring=w359:string, offset past match=w358:i32)  [unwired: 3 out]
          n176 = Match Pattern(string=w353, regular expression="^z" ("Axis ID")) -> (after substring=w354:string, offset past match=w355:i32)  [unwired: 3 out]
          n177 = Match Pattern(string=w353, regular expression="^x" ("Axis ID")) -> (after substring=w362:string, offset past match=w363:i32)  [unwired: 3 out]
          n178 = case shown="1" w358 {
            tunnel: w359 -> [_ w375]
            frame -1, Default {
            }
            frame 1 {
              n179 = Scan From String(input string=w375) -> (output 1=→"By":dbl)  [unwired: 4 in, 3 out]
            }
          }
          n180 = case shown="1" w355 {
            tunnel: w354 -> [_ w373]
            frame -1, Default {
            }
            frame 1 {
              n181 = Scan From String(input string=w373) -> (output 1=→"Bz":dbl)  [unwired: 4 in, 3 out]
            }
          }
          n182 = case shown="1" w363 {
            tunnel: w362 -> [_ w377]
            frame -1, Default {
            }
            frame 1 {
              n183 = Scan From String(input string=w377) -> (output 1=→"Bx":dbl)  [unwired: 4 in, 3 out]
            }
          }
        }
        frame Error {
        }
      }
      n184 = Unbundle(w349) -> ("status"=w348:bool)  [unwired: 2 out]
      n185 = Not(x=w348) -> (.not. x?=→"Соединение":bool)
    }
    n186 = flat-sequence {
      tunnel: [w346] -> w325
      tunnel: w324 -> [w346]
      tunnel: [w345] -> w323
      tunnel: w322 -> [w345]
      frame #0 {
        n187 = Wait (ms)(milliseconds to wait=u32 500) -> ()  [unwired: 1 out]
      }
    }
    n188 = VISA Disable Event ("VISA \nDisable Event")(8:w323, 10:w321, 11:w325) -> (0:w339:errorcluster, 3:w340:refnum<visa-resource-name>)  [unwired: 1 in]
    n189 = VISA Close(VISA resource name=w340, error in (no error)=w339) -> (error out=w338:errorcluster)
    n190 = call <vilib>:"General Error Handler.vi"("type of dialog (OK msg:1)"=w337, "error in (no error)"=w338) -> ("message"=→"String 2":string)  [unwired: 9 in, 4 out]
  }
  "Table num index" <- u32 0 ("Table num index")
